vi "Configure Routing and Faulting Custom Device.vi"() -> ()   [LabVIEW 2017]
uses:
  SubVIs/Routing Channel Configuration.ctl
  NationalInstruments.VeriStand.SystemDefinitionAPI
  SLSC Switch Examples.lvlib
  Routing and Faulting/Scripting/Routing and Faulting Scripting.lvlib
panel:
  in  "Channel Configurations":T1[](array[typedef])=[{"Channel Name"="Window Up", "Initial State"="No Connections", "Description"="Window-Up Sensor State", "State Configurations"=[{"Name"="No Connections", "Description"="no connections", "Value"=-1.0, "Connection List"=[]}, {"Name"="Passthrough", "Description"="sensor connected", "Value"=1.0, "Connection List"=[{"Resource"="SLSC-12001-0314B282-Mod2", "Source"="DUT_Ch0", "Destination"="LOAD_Ch0"}]}, {"Name"="Short to Ground", "Description"="sensor faulted to ground", "Value"=2.0, "Connection List"=[{"Resource"="SLSC-12001-0314B282-Mod2", "Source"="DUT_Ch0", "Destination"="BusA"}]}, {"Name"="Short to Power", "Description"="sensor faulted to power", "Value"=3.0, "Connection List"=[{"Resource"="SLSC-12001-0314B282-Mod2", "Source"="DUT_Ch0", "Destination"="BusB"}]}, {"Name"="Open Circuit", "Description"="open circuit - not connected", "Value"=4.0, "Connection List"=[]}]}, {"Channel Name"="Window Down", "Initial State"="No Connections", "Description"="Window-Up Sensor State", "State Configurations"=[{"Name"="No Connections", "Description"="no connections", "Value"=-1.0, "Connection List"=[]}, {"Name"="Passthrough", "Description"="sensor connected", "Value"=1.0, "Connection List"=[{"Resource"="SLSC-12001-0314B282-Mod2", "Source"="DUT_Ch1", "Destination"="LOAD_Ch1"}]}, {"Name"="Short to Ground", "Description"="sensor faulted to ground", "Value"=2.0, "Connection List"=[{"Resource"="SLSC-12001-0314B282-Mod2", "Source"="DUT_Ch1", "Destination"="BusA"}]}, {"Name"="Short to Power", "Description"="sensor faulted to power", "Value"=3.0, "Connection List"=[{"Resource"="SLSC-12001-0314B282-Mod2", "Source"="DUT_Ch1", "Destination"="BusB"}]}, {"Name"="Open Circuit", "Description"="open circuit - not connected", "Value"=4.0, "Connection List"=[]}]}]
  in  "Output System Definition File":path
  in  "Input System Definition File (Preconfigured with an SLSC custom device)":path
  # "Overview: Demonstrates using the Routing and Faulting custom device scripting API to configure the custom device. \n\nInstructions:\n1. Use one of the SLSC Switch scripting examples (Configure Modules ...) to script one or more SLSC Switch custom devices into a system definition file.\n2. Browse to the system definition created in step 1 to be used as the Input System Definition File.\n3. Browse to a path to save the system definition file as the output Output System Definition File.\n4. For each routing channel you want to configure, use the Channel Configurations array to configure each channel's Name and Description.\n5. For each State, use the State Configurations array to set the State Name, Value, Description, and Connections List.\n6. For each Connection, set the connection Resource, Source endpoint, and Destination endpoint.\n7. After configurating each State, set the routing channel's Initial State (initial set of connections on deployment).\n8. Repeat steps 4-7. for each routing channel in your custom device.\n9. Run the VI and verify its results."
  # "System Definition Files"
  # "Routing and Faulting Custom Device Configuration"
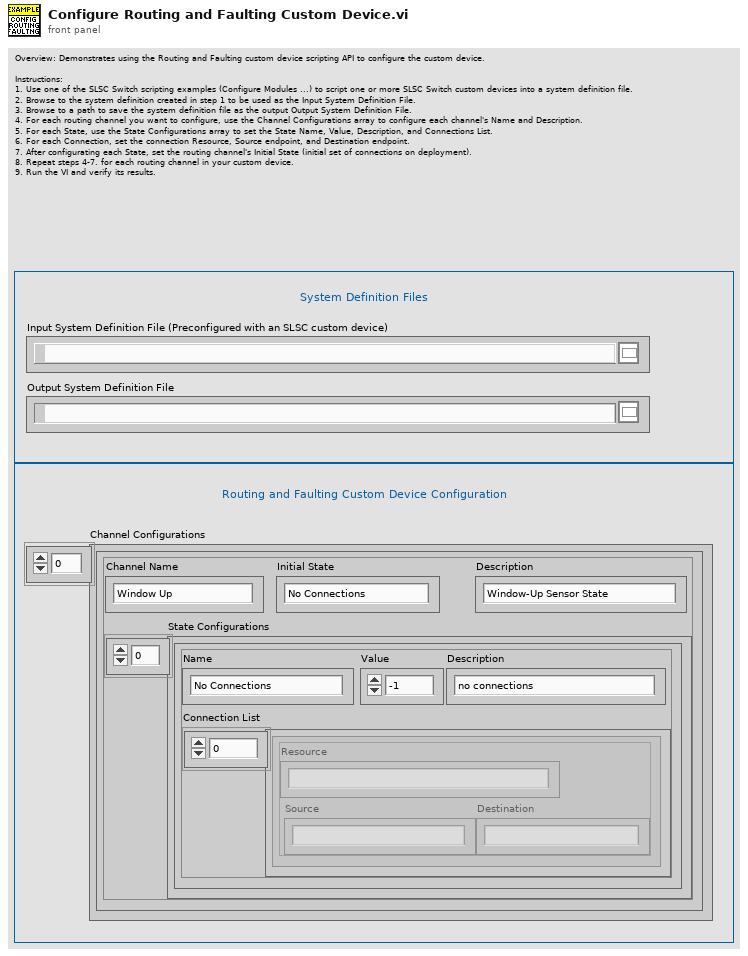
[diagram p1: front panel]
types:
  T1 = typedef "SLSC Switch Examples.lvlib/Routing Channel Configuration.ctl" = cluster{"Channel Name":string, "Initial State":string, "Description":string, "State Configurations":cluster{"Name":string, "Description":string, "Value":dbl, "Connection List":cluster{"Resource":string, "Source":string, "Destination":string}[]}[]}
  T2 = typedef "Custom Device API.lvlib/Custom Device Item Ref.ctl" = u64
  T3 = cluster{"Name":string, "Description":string, "Value":dbl, "Connection List":cluster{"Resource":string, "Source":string, "Destination":string}[]}[]
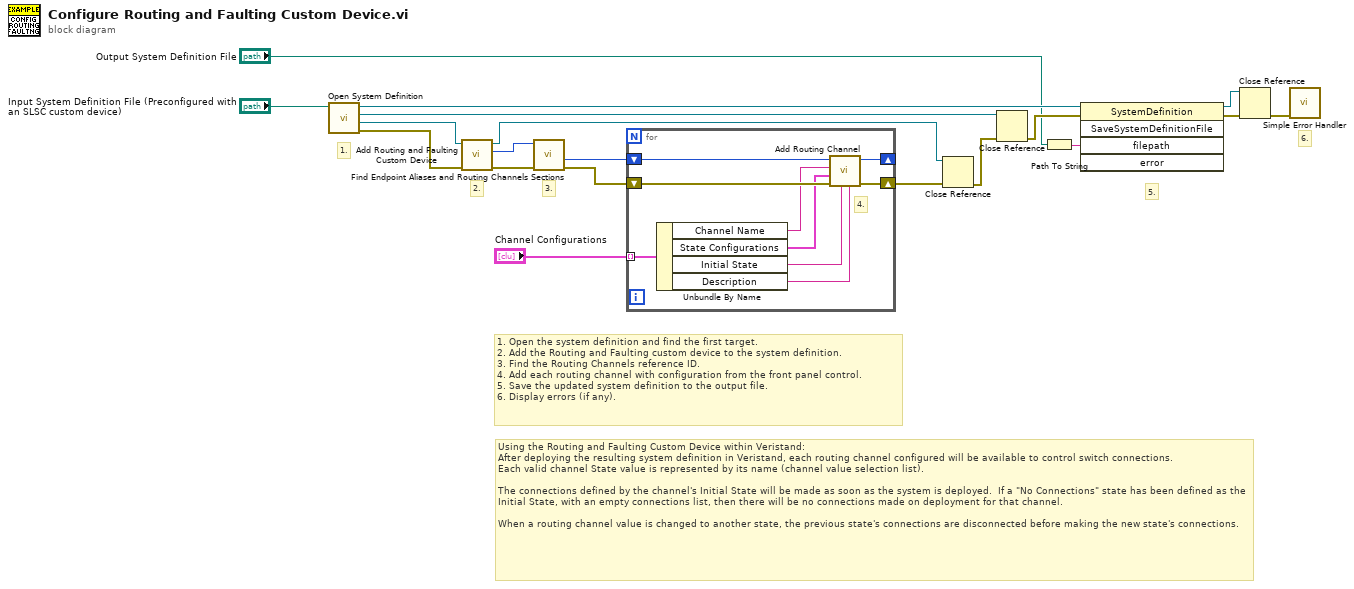
[diagram p0: block diagram]
diagram:
  # "Using the Routing and Faulting Custom Device within Veristand:\nAfter deploying the resulting system definition in Veristand, each routing channel configured will be available to control switch connections.\nEach valid channel State value is represented by its name (channel value selection list).\n\nThe connections defined by the channel's Initial State will be made as soon as the system is deployed.  If a \"No Connections\" state has been defined as the Initial State, with an empty connections list, then there will be no connections made on deployment for that channel.\n\nWhen a routing channel value is changed to another state, the previous state's connections are disconnected before making the new state's connections."
  # "3."
  # "2."
  # "5."
  # "6."
  # "8."
  # "1."
  # "1. Open the system definition and find the first target.\n2. Add the Routing and Faulting custom device to the system definition.\n3. Find the Routing Channels reference ID.\n4. Add each routing channel with configuration from the front panel control.\n5. Save the updated system definition to the output file.\n6. Display errors (if any)."
  n1 = call "Open System Definition.vi"("System Definition File"="Input System Definition File (Preconfigured with an SLSC custom device)") -> ("error out"=w1:errorcluster, "Target Refnum"=w9:refnum<k24>, "Root Refnum"=w15:refnum<k24>, "System Definition Refnum"=w19:refnum<k24>)  [unwired: 7 in]
  n2 = call "Add Routing and Faulting Custom Device.vi"("error in (no error)"=w1, "Target in"=w9) -> ("error out"=w7:errorcluster, "Routing and Faulting Custom Device Ref"=w8:T2, "Target out"=w6:refnum<k24>)  [unwired: 7 in]
  n3 = call "Find Endpoint Aliases and Routing Channels Sections.vi"("error in (no error)"=w7, "Routing and Faulting Custom Device Ref in"=w8) -> ("error out"=w5:errorcluster, "Routing Channels Ref"=w4:T2)  [unwired: 6 in, 2 out]
  n4 = for {
    shift-right: [w26] -> w3
    shift-left: w5 -> [w28]
    shift-right: [w25] -> _
    shift-left: w4 -> [w27]
    tunnel: "Channel Configurations" -> [w24] mode=indexing
    # "4."
    n5 = Unbundle By Name(w24) -> ("Channel Name"=w22:string, "State Configurations"=w23:T3, "Initial State"=w21:string, "Description"=w20:string)
    n6 = call "Add Routing Channel.vi"("Description"=w20, "Initial State"=w21, "error in (no error)"=w28, "State Configurations"=w23, "Channel Name"=w22, "Routing Channels Ref in"=w27) -> ("error out"=w26:errorcluster, "Routing Channels Ref out"=w25:T2)  [unwired: 3 in, 1 out]
  }
  n7 = Close Reference(reference=w6, error in (no error)=w3) -> (error out=w12:errorcluster)
  n8 = Close Reference(reference=w15, error in (no error)=w12) -> (error out=w14:errorcluster)
  n9 = Path To String(path="Output System Definition File") -> (string=w18:string)
  n10 = invoke class="SystemDefinition" method="SaveSystemDefinitionFile"(reference=w19, error in=w14, "filepath"=w18) -> (reference out=w16:refnum<k24>, error out=w17:errorcluster)  [unwired: 2 in, 3 out]
  n11 = Close Reference(reference=w16, error in (no error)=w17) -> (error out=w11:errorcluster)
  n12 = call <vilib>:"Simple Error Handler.vi"("error in (no error)"=w11) -> ()  [unwired: 1 in, 8 out]
